vi "SSL Detection Frame Simple Estimator Cameras.vi"(5 "Estimador":T1, 7 "Enable":bool, 8 "ignora esquerda?":bool=TRUE, 9 "ignora lado?":bool=TRUE, 10 "Field Size":T2, 11 "Detection Frame In":T3 {"robots_blue"."height" format="%+4.3f"; "robots_blue"."pixel_y" format="%+4.3f"; "robots_blue"."pixel_x" format="%+4.3f"; "robots_blue"."orientation" format="%+4.3f"; "robots_blue"."y" format="%+4.3f"; "robots_blue"."confidence" format="%4.3f"; "robots_blue"."x" format="%+4.3f"; "robots_yellow"."height" format="%+4.3f"; "robots_yellow"."pixel_y" format="%+4.3f"; "robots_yellow"."pixel_x" format="%+4.3f"; "robots_yellow"."orientation" format="%+4.3f"; "robots_yellow"."y" format="%+4.3f"; "robots_yellow"."confidence" format="%4.3f"; "robots_yellow"."x" format="%+4.3f"}) -> (2 "Field Size Out":T2, 3 "Detection Frame Out":T3 {"robots_blue"."height" format="%+4.3f"; "robots_blue"."pixel_y" format="%+4.3f"; "robots_blue"."pixel_x" format="%+4.3f"; "robots_blue"."orientation" format="%+4.3f"; "robots_blue"."y" format="%+4.3f"; "robots_blue"."confidence" format="%4.3f"; "robots_blue"."x" format="%+4.3f"; "robots_yellow"."height" format="%+4.3f"; "robots_yellow"."pixel_y" format="%+4.3f"; "robots_yellow"."pixel_x" format="%+4.3f"; "robots_yellow"."orientation" format="%+4.3f"; "robots_yellow"."y" format="%+4.3f"; "robots_yellow"."confidence" format="%4.3f"; "robots_yellow"."x" format="%+4.3f"})   [LabVIEW 2017]
uses:
  SSL Detection Robot.ctl
  SSL Detection Ball.ctl
  SSL Detection Frame.ctl
  <vilib>/Analysis/Matrix/Datatypes/RealMatrix.ctl
  <vilib>/Analysis/Matrix/NI_Matrix.lvlib
  Filters/Estimadores.ctl
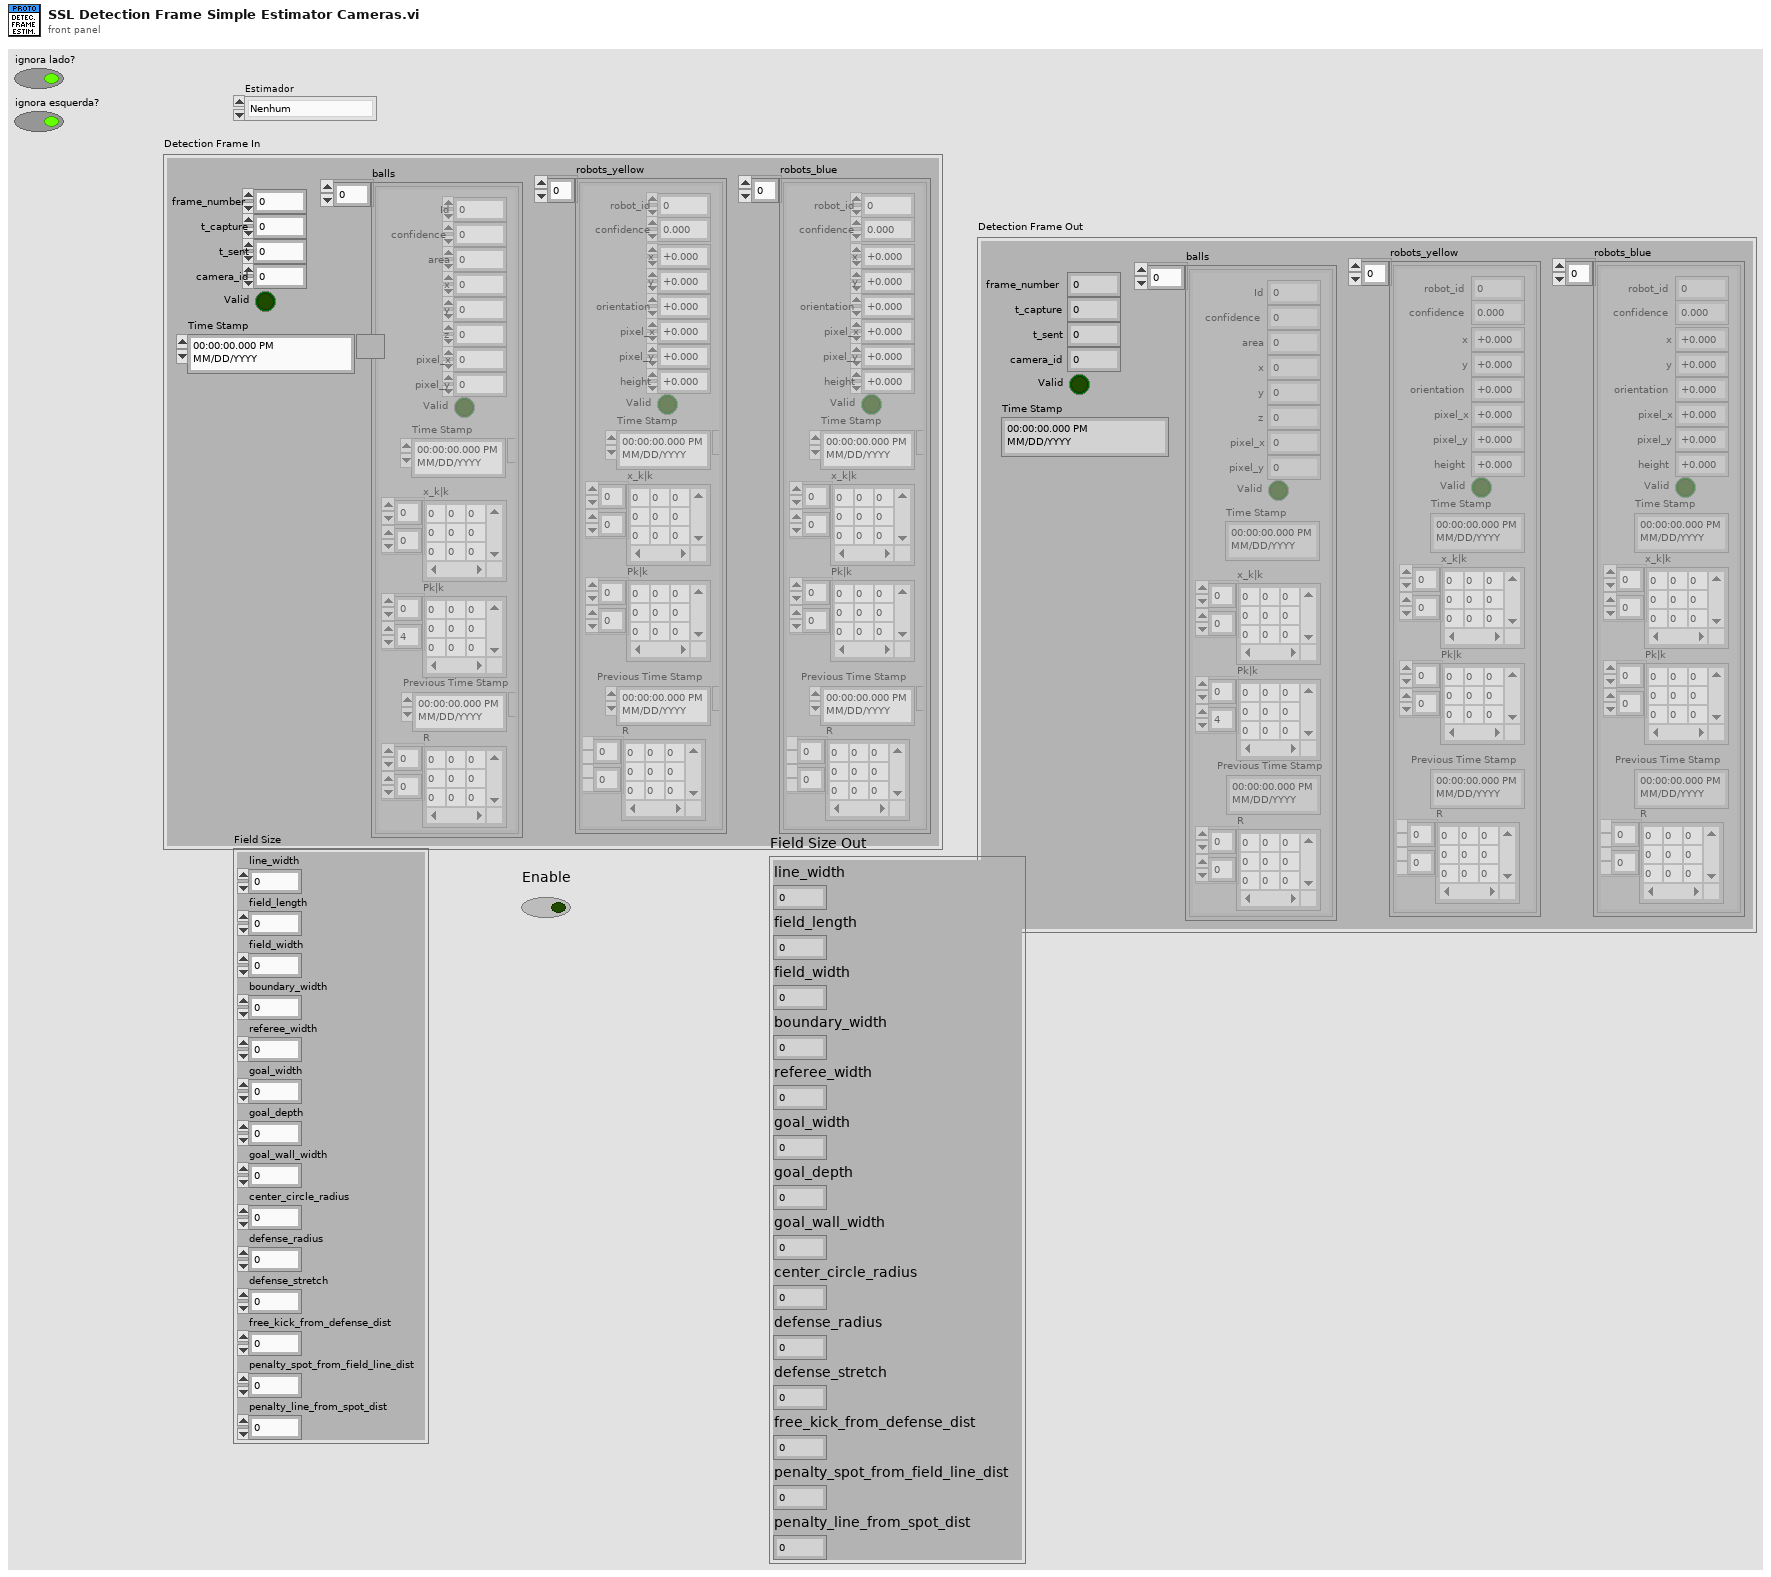
[diagram p1: front panel]
types:
  T1 = typedef "Estimadores.ctl" = enum16{"Nenhum", "Simples", "Kalman"}
  T2 = cluster{"line_width":u32, "field_length":u32, "field_width":u32, "boundary_width":u32, "referee_width":u32, "goal_width":u32, "goal_depth":u32, "goal_wall_width":u32, "center_circle_radius":u32, "defense_radius":u32, "defense_stretch":u32, "free_kick_from_defense_dist":u32, "penalty_spot_from_field_line_dist":u32, "penalty_line_from_spot_dist":u32}
  T3 = typedef "SSL Detection Frame.ctl" = cluster{"frame_number":u32, "t_capture":dbl, "t_sent":dbl, "camera_id":u32, "robots_yellow":T4[], "robots_blue":T4[], "balls":T6[], "Valid":bool, "Time Stamp":timestamp}
  T4 = typedef "SSL Detection Robot.ctl" = cluster{"x":sgl, "robot_id":u32, "confidence":sgl, "y":sgl, "orientation":sgl, "pixel_x":sgl, "pixel_y":sgl, "height":sgl, "Valid":bool, "Time Stamp":timestamp, "x_k|k":T5, "Pk|k":T5, "Previous Time Stamp":timestamp, "R":T5}
  T5 = typedef "NI_Matrix.lvlib/RealMatrix.ctl" = dbl[][]
  T6 = typedef "SSL Detection Ball.ctl" = cluster{"x":sgl, "area":u32, "confidence":sgl, "y":sgl, "z":sgl, "pixel_x":sgl, "pixel_y":sgl, "Valid":bool, "Time Stamp":timestamp, "x_k|k":T5, "Pk|k":T5, "Id":u32, "Previous Time Stamp":timestamp, "R":T5}
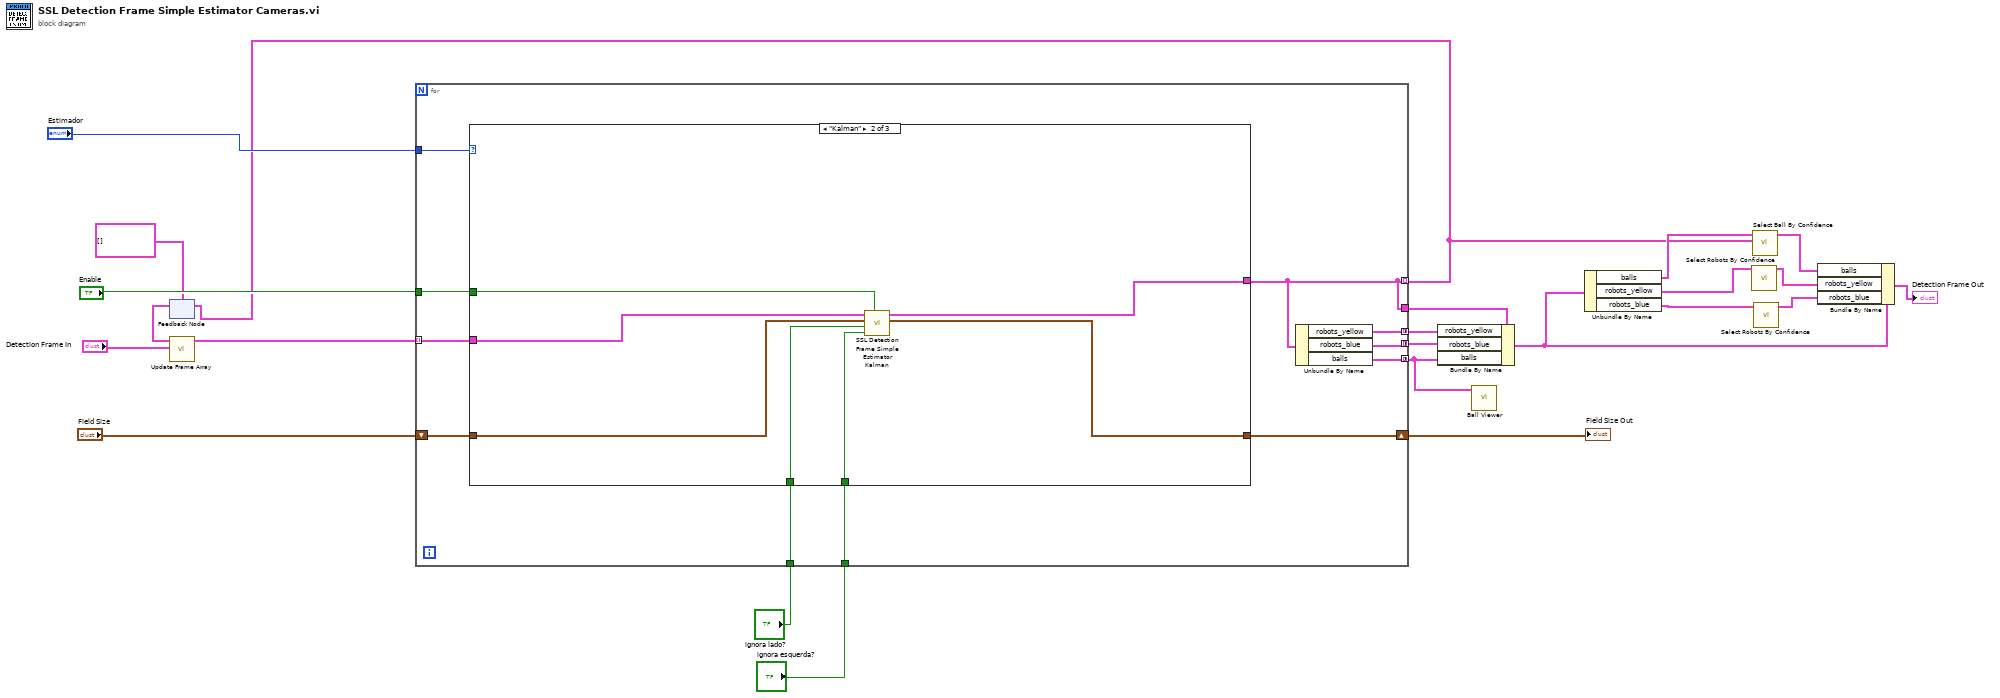
[diagram p0: block diagram]
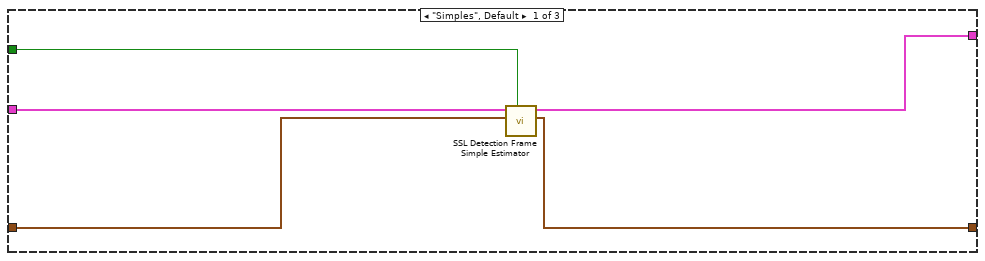
[diagram p2: hidden frame]
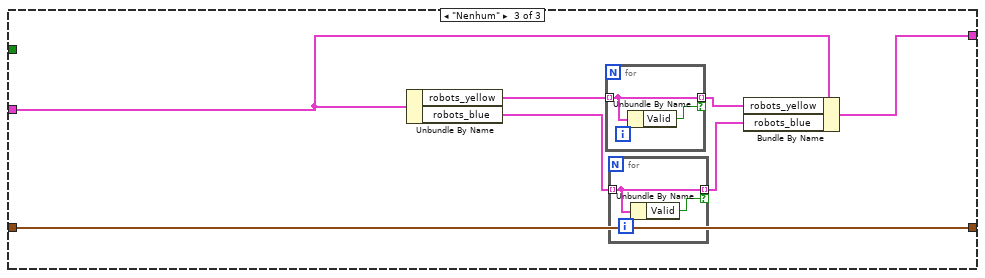
[diagram p3: hidden frame]
diagram:
  n1 = feedback #1(T3[] [] ("Detection Frame In out")) -> (w19:T3[])
  n2 = call "Update Frame Array.vi"("Detection Frame In"="Detection Frame In", "Detection Frame In 2"=w19) -> ("Detection Frame In out"=w20:T3[])  [unwired: 9 in]
  n3 = for {
    tunnel: [w26] -> w1 mode=indexing
    tunnel: "Estimador" -> [w32]
    tunnel: "Enable" -> [w31]
    tunnel: w20 -> [w30] mode=indexing
    shift-right: [w33] -> w22
    shift-left: "Field Size" -> [w34]
    tunnel: [w29] -> w16 mode=concatenating
    tunnel: [w28] -> w15 mode=concatenating
    tunnel: [w27] -> w4 mode=concatenating
    tunnel: [w26] -> w17
    tunnel: "ignora lado?" -> [w25]
    tunnel: "ignora esquerda?" -> [w24]
    n4 = case shown="\"Kalman\"" w32 {
      tunnel: [w35 w45 w49] -> w26
      tunnel: w30 -> [w39 w46 w51]
      tunnel: w31 -> [w38 w42 _]
      tunnel: w34 -> [w37 w44 w53]
      tunnel: [w36 w43 w53] -> w33
      tunnel: w25 -> [_ w41 _]
      tunnel: w24 -> [_ w40 _]
      frame "Simples", Default {
        n5 = call "SSL Detection Frame Simple Estimator.vi"("Enable"=w38, "Field Size"=w37, "Detection Frame In"=w39) -> ("Field Size Out"=w36:T2, "Detection Frame Out"=w35:T3)  [unwired: 7 in]
      }
      frame "Kalman" {
        n6 = call "SSL Detection Frame Simple Estimator Kalman.vi"("Enable"=w42, "ignora esquerda?"=w40, "ignora lado?"=w41, "Field Size"=w44, "Detection Frame In"=w46) -> ("Field Size Out"=w43:T2, "Detection Frame Out"=w45:T3)  [unwired: 5 in]
      }
      frame "Nenhum" {
        n7 = Unbundle By Name(w51) -> ("robots_yellow"=w52:T4[], "robots_blue"=w48:T4[])
        n8 = for {
          tunnel: w52 -> [w57] mode=indexing
          tunnel: [w57] -> w50 mode=indexing if=w56
          n9 = Unbundle By Name(w57) -> ("Valid"=w56:bool)
        }
        n10 = for {
          tunnel: w48 -> [w55] mode=indexing
          tunnel: [w55] -> w47 mode=indexing if=w54
          n11 = Unbundle By Name(w55) -> ("Valid"=w54:bool)
        }
        n12 = Bundle By Name(cluster=w51, "robots_yellow"=w50, "robots_blue"=w47) -> (w49:T3)
      }
    }
    n13 = Unbundle By Name(w26) -> ("robots_yellow"=w29:T4[], "robots_blue"=w28:T4[], "balls"=w27:T6[])
  }
  "Field Size Out" <- w22
  n14 = feedback-in #1(w1) -> ()
  n15 = Bundle By Name(cluster=w17, "robots_yellow"=w16, "robots_blue"=w15, "balls"=w4) -> (w12:T3)
  n16 = call "Ball Viewer.vi"("balls"=w4) -> ()  [unwired: 11 in]
  n17 = Unbundle By Name(w12) -> ("balls"=w3:T6[], "robots_yellow"=w8:T4[], "robots_blue"=w13:T4[])
  n18 = call "Select Robots By Confidence.vi"("robots_blue"=w8) -> ("Array"=w7:T4[])  [unwired: 10 in]
  n19 = call "Select Ball By Confidence.vi"("Array"=w1, "balls"=w3) -> ("balls out"=w2:T6[])  [unwired: 9 in]
  n20 = call "Select Robots By Confidence.vi"("robots_blue"=w13) -> ("Array"=w11:T4[])  [unwired: 10 in]
  n21 = Bundle By Name(cluster=w12, "balls"=w2, "robots_yellow"=w7, "robots_blue"=w11) -> (→"Detection Frame Out":T3)
